vi "DequeueCmd_WithHold.vi"(8 "error in (no error)":errorcluster, 10 "Timeout (ms)":i32=-1, 11 "Queue In":T1) -> (0 "error out":errorcluster, 1 "arguments":string[](array[string]), 2 "command":string="Default", 3 "queue (dup)":T1, 5 "Data":variant)   [LabVIEW 2010]
doc: "This VI serves to dequeue a command from the string queue provided to the input. The queue sorts the command from the command line arguements, which can be included after the command. The arguements are separated by a colon (:) and will be output as a string array. The VI will also handle any error that exists in the error cluster by setting the command = Error with the error code and error string message as arguments.\n\nInputs:\nqueue - input queue (string)\nTimeout (ms) - timeout (in milliseconds) for the dequeue function to wait (default -1 = no timeout)\nerror in - error input cluster\n\nOutputs:\ncommand - main state in the queue; this is used as the current state to be used by the case structure\narguments - command line arguments that were included with the command; separated by colon (:)\nqueue - duplicate reference for the queue\nerror out - error output cluster"
uses:
  <userlib>/Common/Queue with Cluster/TYP_Queue with Cluster Reference.ctl
  <userlib>/Common/Queue with Cluster/Enqueue - ClusterBoth.vi
panel:
  # "Inputs"
  # "Outputs"
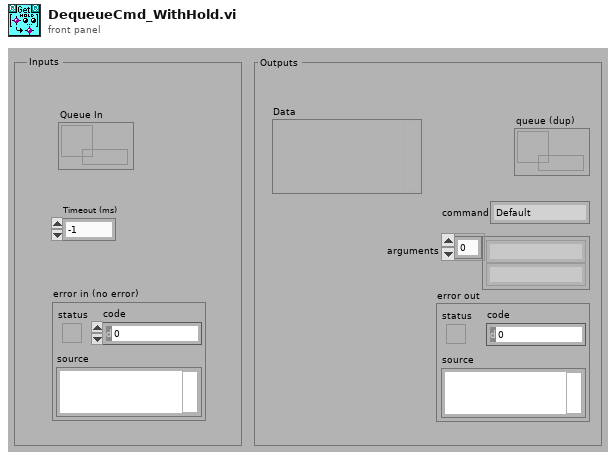
[diagram p1: front panel]
types:
  T1 = typedef "TYP_Queue with Cluster Reference.ctl" = refnum<queue>
  T2 = typedef "TYP_Queue Cluster Element.ctl" = cluster{"Command":string, "Data":variant}
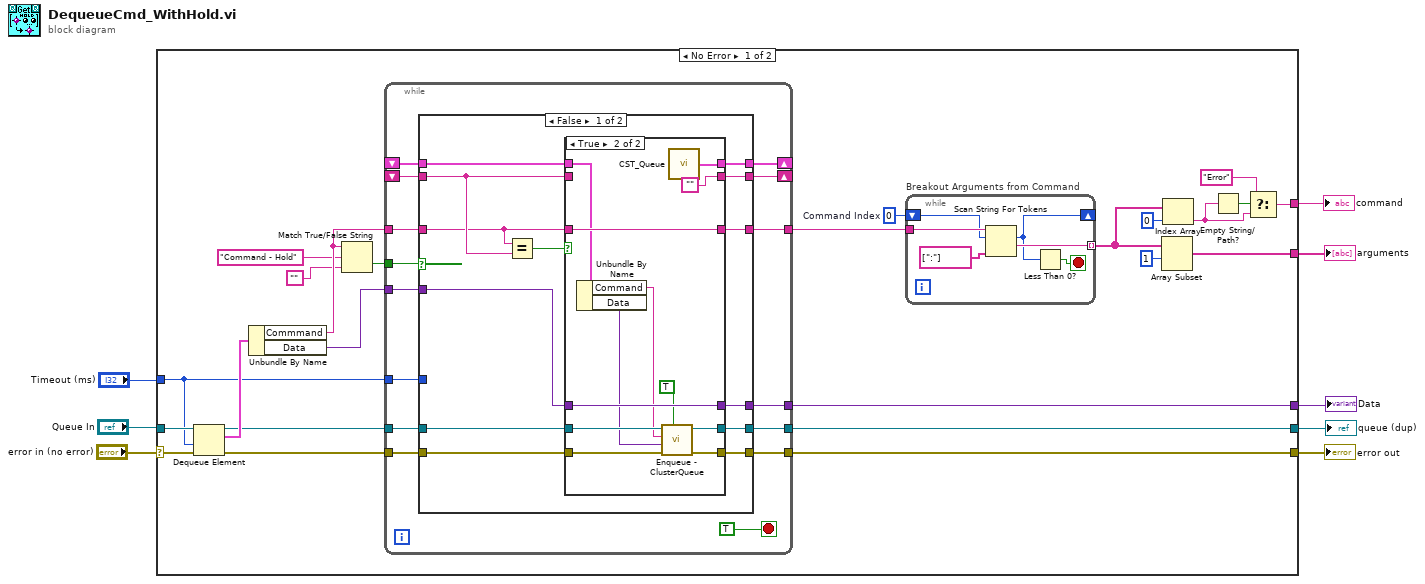
[diagram p0: block diagram]
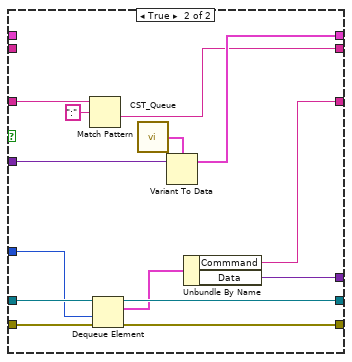
[diagram p3: hidden frame]
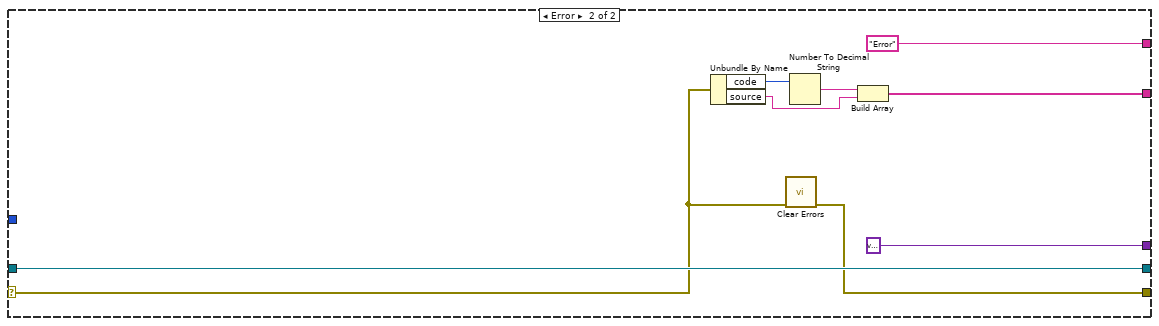
[diagram p4: hidden frame]
diagram:
  n1 = case shown="No Error" "error in (no error)" {
    selector: "error in (no error)" -> [w29 w102]
    tunnel: [w14 w101] -> w8
    tunnel: "Queue In" -> [w32 w107]
    tunnel: [w31 w104] -> w7
    tunnel: [w15 w107] -> w3
    tunnel: [w30 "Error" ("token string")] -> w6
    tunnel: [w16 variant ("Data")] -> w2
    tunnel: "Timeout (ms)" -> [w13 _]
    frame No Error {
      w27 = 0  # Command Index
      n2 = Dequeue Element(queue=w32, timeout in ms (-1)=w13, error in (no error)=w29) -> (queue out=w19:T1, element=w28:cluster{"Commmand":string, "Data":variant}, error out=w18:errorcluster)  [unwired: 1 out]
      n3 = Unbundle By Name(w28) -> ("Commmand"=w12:string, "Data"=w17:variant)
      n4 = Match True/False String(2:"", 3:"Command - Hold" ("y"), 4:w12) -> (0:w10:bool)  [unwired: 1 out]
      n5 = while {
        tunnel: w10 -> [w33]
        tunnel: [w46] -> w20
        tunnel: w12 -> [w45]
        tunnel: w17 -> [w44]
        tunnel: w19 -> [w43]
        tunnel: w18 -> [w42]
        shift-right: [w41] -> _
        shift-left: _ -> [w40]
        tunnel: [w39] -> w16
        tunnel: [w38] -> w15
        tunnel: [w37] -> w14
        tunnel: w13 -> [w36]
        shift-right: [w35] -> _
        shift-left: _ -> [w34]
        stop <- TRUE stop-if-true
        n6 = case shown="False" w33 {
          tunnel: [w50 w84] -> w46
          tunnel: w45 -> [w51 w81]
          tunnel: w44 -> [w49 w92]
          tunnel: w43 -> [w59 w91]
          tunnel: w42 -> [w60 w90]
          tunnel: [w53 w89] -> w41
          tunnel: w40 -> [w54 _]
          tunnel: [w48 w83] -> w39
          tunnel: [w58 w87] -> w38
          tunnel: [w57 w86] -> w37
          tunnel: w36 -> [_ w88]
          tunnel: [w52 w79] -> w35
          tunnel: w34 -> [w55 _]
          frame False {
            n7 = Equal?(x=w51, y=w55) -> (x = y?=w56:bool)
            n8 = case shown="True" w56 {
              tunnel: w60 -> [w62 w68]
              tunnel: w59 -> [w63 w78]
              tunnel: [w63 w77] -> w58
              tunnel: [w62 w76] -> w57
              tunnel: w55 -> [w65 _]
              tunnel: w54 -> [w66 w70]
              tunnel: [w66 w73] -> w53
              tunnel: [w65 ""] -> w52
              tunnel: w51 -> [w64 w75]
              tunnel: [w64 w75] -> w50
              tunnel: w49 -> [w61 w74]
              tunnel: [w61 w74] -> w48
              frame False {
              }
              frame True {
                n9 = Unbundle By Name(w70) -> ("Command"=w69:string, "Data"=w67:variant)
                n10 = call-poly <userlib>:"Enqueue - ClusterQueue.vi"("At Front? (F)"=TRUE, "error in (no error)"=w68, "Data"=w67, "Command"=w69, "Queue with Cluster Reference"=w78) -> ("error out"=w76:errorcluster, "Queue Out (dup)"=w77:T1)  [unwired: 5 in]
                n11 = call <userlib>:"CST_Queue.vi"() -> ("Queue Cluster Element"=w73:T2)  [unwired: 1 in]
              }
            }
          }
          frame True {
            n12 = Match Pattern(string=w81, regular expression=":") -> (after substring=w79:string)  [unwired: 1 in, 3 out]
            n13 = Dequeue Element(queue=w91, timeout in ms (-1)=w88, error in (no error)=w90) -> (queue out=w87:T1, element=w85:cluster{"Commmand":string, "Data":variant}, error out=w86:errorcluster)  [unwired: 1 out]
            n14 = call <userlib>:"CST_Queue.vi"() -> ("Queue Cluster Element"=w82:T2)  [unwired: 1 in]
            n15 = Variant To Data(Variant=w92, type=w82) -> (data=w89:T2)  [unwired: 1 in, 1 out]
            n16 = Unbundle By Name(w85) -> ("Commmand"=w84:string, "Data"=w83:variant)
          }
        }
      }
      n17 = while "Breakout Arguments from Command" {
        tunnel: [w98] -> w25 mode=indexing
        tunnel: w20 -> [w96]
        shift-right: [w95] -> _
        shift-left: w27 -> [w94]
        stop <- w97 stop-if-true
        n18 = Scan String For Tokens(6:string[] [":"] ("delimiters (\\s,\\t,\\r,\\n)"), 8:w94, 9:w96) -> (1:w98:string, 2:w95:i32)  [unwired: 3 in, 2 out]
        n19 = Less Than 0?(x=w95) -> (x < 0?=w97:bool)
      }
      n20 = Array Subset(array=w25, index=1) -> (w31:string[])  [unwired: 1 in]
      n21 = Index Array(array=w25, index=0) -> (element=w22:string)
      n22 = Empty String/Path?(string/path=w22) -> (empty?=w23:bool)
      n23 = Select(t="Error", s=w23, f=w22) -> (s? t:f=w30:string)
    }
    frame Error {
      n24 = Unbundle By Name(w102) -> ("code"=w105:i32, "source"=w100:string)
      n25 = call <vilib>:"Clear Errors.vi"("error in (no error)"=w102) -> ("error out"=w101:errorcluster)  [unwired: 6 in]
      n26 = Number To Decimal String(number=w105) -> (decimal integer string=w103:string)  [unwired: 1 in]
      n27 = Build Array(w103, w100) -> (w104:string[])
    }
  }
  "error out" <- w8
  "arguments" <- w7
  "command" <- w6
  "queue (dup)" <- w3
  "Data" <- w2
